vi "Global 1.vi"() -> ()   [LabVIEW 2020]
panel:
  in  "Boton1":bool
  in  "stop":bool
  out "Numero a pasar":i32
  out "LED1":bool=TRUE
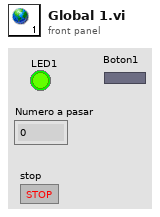
[diagram p1: front panel]
diagram:
